vi "App - analyze RUS V6.vi"() -> ()   [LabVIEW 2021] (continued)
"z center"=0.03600000000000003+0.0040000000000000036i, "z(0)"=-0.1817049418249758+0.4229026946079033i, "radius"=0.47209629234381667}}, "timestamp(min)"=320.0, "timestamp"=timestamp(3493747021 s since 1904-01-01), "Magn Field(T)"=0.0}, {"temperature"=155.917, "lorentzian"={"A (VHz)"=0.0003600783098296233, "ω (Hz)"=667.5871571554018, "Γ (Hz)"=0.0666645074516891, "φ (rad)"=3.6415323231958747, "Q"=10014.131697278248, "Norm  Ampl"=0.03138403226728406, "z∞ (V)"=0.2616769830982948-0.40115818854601326i, "4corners"={"z (-pi/2)"=-0.37715818854601324-0.21367698309829475i, "z(inf)"=0.2616769830982948-0.40115818854601326i, "z (pi/2)"=0.4491581885460133+0.23767698309829477i, "z center"=0.03600000000000003+0.01200000000000001i, "z(0)"=-0.18967698309829473+0.4251581885460133i, "radius"=0.4707757315994221}}, "timestamp(min)"=321.33333333581686, "timestamp"=timestamp(3493747101 s since 1904-01-01), "Magn Field(T)"=0.0}, {"temperature"=155.569, "lorentzian"={"A (VHz)"=0.0003591126324986569, "ω (Hz)"=667.603372353538, "Γ (Hz)"=0.06609971655941053, "φ (rad)"=3.6523793327906917, "Q"=10099.943042168645, "Norm  Ampl"=0.03138978061501275, "z∞ (V)"=0.2681541455231212-0.4022709936013601i, "4corners"={"z (-pi/2)"=-0.3782709936013601-0.22015414552312118i, "z(inf)"=0.2681541455231212-0.4022709936013601i, "z (pi/2)"=0.45027099360136014+0.2441541455231212i, "z center"=0.03600000000000003+0.01200000000000001i, "z(0)"=-0.19615414552312116+0.4262709936013601i, "radius"=0.47488525290119155}}, "timestamp(min)"=322.6499999985099, "timestamp"=timestamp(3493747180 s since 1904-01-01), "Magn Field(T)"=0.0}, {"temperature"=155.24, "lorentzian"={"A (VHz)"=0.0003558702433597225, "ω (Hz)"=667.6196504795548, "Γ (Hz)"=0.06570935152346731, "φ (rad)"=3.666739520729764, "Q"=10160.192347068323, "Norm  Ampl"=0.03117556747840149, "z∞ (V)"=0.27385901621365416-0.39851492868577315i, "4corners"={"z (-pi/2)"=-0.37451492868577313-0.22585901621365412i, "z(inf)"=0.27385901621365416-0.39851492868577315i, "z (pi/2)"=0.4465149286857732+0.24985901621365414i, "z center"=0.03600000000000003+0.01200000000000001i, "z(0)"=-0.2018590162136541+0.4225149286857732i, "radius"=0.47444643350752763}}, "timestamp(min)"=323.9666666686535, "timestamp"=timestamp(3493747259 s since 1904-01-01), "Magn Field(T)"=0.0}, {"temperature"=154.892, "lorentzian"={"A (VHz)"=0.0003530566967995145, "ω (Hz)"=667.6345004307237, "Γ (Hz)"=0.06544080329072241, "φ (rad)"=3.6774068000638085, "Q"=10202.11346527549, "Norm  Ampl"=0.03099707161072482, "z∞ (V)"=0.27782594111484155-0.3952830971115466i, "4corners"={"z (-pi/2)"=-0.37128309711154656-0.2298259411148415i, "z(inf)"=0.27782594111484155-0.3952830971115466i, "z (pi/2)"=0.4432830971115466+0.2538259411148415i, "z center"=0.03600000000000003+0.01200000000000001i, "z(0)"=-0.20582594111484148+0.4192830971115466i, "radius"=0.4736658178387504}}, "timestamp(min)"=325.30000000447035, "timestamp"=timestamp(3493747339 s since 1904-01-01), "Magn Field(T)"=0.0}, {"temperature"=154.55, "lorentzian"={"A (VHz)"=0.00035235220794812265, "ω (Hz)"=667.6414584582035, "Γ (Hz)"=0.06583438070884551, "φ (rad)"=3.6599783805757107, "Q"=10141.227900523096, "Norm  Ampl"=0.031187058102442655, "z∞ (V)"=0.262718083957458-0.39948267452777714i, "4corners"={"z (-pi/2)"=-0.3834826745277771-0.22271808395745793i, "z(inf)"=0.262718083957458-0.39948267452777714i, "z (pi/2)"=0.4394826745277772+0.24671808395745795i, "z center"=0.028000000000000025+0.01200000000000001i, "z(0)"=-0.20671808395745792+0.42348267452777716i, "radius"=0.4737199281993453}}, "timestamp(min)"=326.6166666671634, "timestamp"=timestamp(3493747418 s since 1904-01-01), "Magn Field(T)"=0.0}, {"temperature"=154.223, "lorentzian"={"A (VHz)"=0.0003545258955251594, "ω (Hz)"=667.6596980423662, "Γ (Hz)"=0.06596121803706546, "φ (rad)"=3.6664657392703672, "Q"=10122.003776024716, "Norm  Ampl"=0.03132255223514789, "z∞ (V)"=0.2739554373795724-0.40694066198896567i, "4corners"={"z (-pi/2)"=-0.37494066198896564-0.23395543737957233i, "z(inf)"=0.2739554373795724-0.40694066198896567i, "z (pi/2)"=0.4469406619889657+0.24195543737957234i, "z center"=0.03600000000000003+0.0040000000000000036i, "z(0)"=-0.2019554373795723+0.4149406619889657i, "radius"=0.47486315697728426}}, "timestamp(min)"=327.95000000298023, "timestamp"=timestamp(3493747498 s since 1904-01-01), "Magn Field(T)"=0.0}, {"temperature"=153.877, "lorentzian"={"A (VHz)"=0.0003464844794787016, "ω (Hz)"=667.6762506062214, "Γ (Hz)"=0.06468629451459908, "φ (rad)"=3.686205850400607, "Q"=10321.757578114684, "Norm  Ampl"=0.030601207625047026, "z∞ (V)"=0.2810920510849647-0.3926307234080894i, "4corners"={"z (-pi/2)"=-0.3686307234080894-0.2330920510849647i, "z(inf)"=0.2810920510849647-0.3926307234080894i, "z (pi/2)"=0.44063072340808945+0.2570920510849647i, "z center"=0.03600000000000003+0.01200000000000001i, "z(0)"=-0.20909205108496468+0.41663072340808943i, "radius"=0.47307096278548816}}, "timestamp(min)"=329.26666666567326, "timestamp"=timestamp(3493747577 s since 1904-01-01), "Magn Field(T)"=0.0}, {"temperature"=153.533, "lorentzian"={"A (VHz)"=0.00034529942679625386, "ω (Hz)"=667.6919916866713, "Γ (Hz)"=0.06439844993865426, "φ (rad)"=3.697376351094415, "Q"=10368.137623230254, "Norm  Ampl"=0.030502173386016206, "z∞ (V)"=0.28590085026076295-0.3903576087759872i, "4corners"={"z (-pi/2)"=-0.36635760877598716-0.2379008502607629i, "z(inf)"=0.28590085026076295-0.3903576087759872i, "z (pi/2)"=0.43835760877598723+0.26190085026076293i, "z center"=0.03600000000000003+0.01200000000000001i, "z(0)"=-0.2139008502607629+0.4143576087759872i, "radius"=0.47364763305751106}}, "timestamp(min)"=330.58333333581686, "timestamp"=timestamp(3493747656 s since 1904-01-01), "Magn Field(T)"=0.0}, {"temperature"=153.206, "lorentzian"={"A (VHz)"=0.00034827333081709075, "ω (Hz)"=667.704330610667, "Γ (Hz)"=0.0656929969706585, "φ (rad)"=3.67323809413097, "Q"=10164.010798729341, "Norm  Ampl"=0.03128951043987482, "z∞ (V)"=0.2774609121600786-0.4065574132803119i, "4corners"={"z (-pi/2)"=-0.3745574132803119-0.23746091216007859i, "z(inf)"=0.2774609121600786-0.4065574132803119i, "z (pi/2)"=0.44655741328031195+0.2454609121600786i, "z center"=0.03600000000000003+0.0040000000000000036i, "z(0)"=-0.20546091216007856+0.4145574132803119i, "radius"=0.4762990255087638}}, "timestamp(min)"=331.91666666418314, "timestamp"=timestamp(3493747736 s since 1904-01-01), "Magn Field(T)"=0.0}, {"temperature"=152.863, "lorentzian"={"A (VHz)"=0.0003372130117361326, "ω (Hz)"=667.7178274337781, "Γ (Hz)"=0.06419396759064425, "φ (rad)"=3.6582012443053293, "Q"=10401.566572294132, "Norm  Ampl"=0.03048428381427238, "z∞ (V)"=0.2625583169568325-0.40090583410884956i, "4corners"={"z (-pi/2)"=-0.38490583410884954-0.2225583169568325i, "z(inf)"=0.2625583169568325-0.40090583410884956i, "z (pi/2)"=0.4409058341088496+0.24655831695683253i, "z center"=0.028000000000000025+0.01200000000000001i, "z(0)"=-0.2065583169568325+0.4249058341088496i, "radius"=0.47487770203995333}}, "timestamp(min)"=333.23333333432674, "timestamp"=timestamp(3493747815 s since 1904-01-01), "Magn Field(T)"=0.0}, {"temperature"=152.533, "lorentzian"={"A (VHz)"=0.0003397272875597955, "ω (Hz)"=667.7315679125422, "Γ (Hz)"=0.06505456301107017, "φ (rad)"=3.657146799356104, "Q"=10264.17728451909, "Norm  Ampl"=0.030891975244662705, "z∞ (V)"=0.2701153266514513-0.409139744947861i, "4corners"={"z (-pi/2)"=-0.37713974494786096-0.23011532665145132i, "z(inf)"=0.2701153266514513-0.409139744947861i, "z (pi/2)"=0.449139744947861+0.23811532665145133i, "z center"=0.03600000000000003+0.0040000000000000036i, "z(0)"=-0.1981153266514513+0.417139744947861i, "radius"=0.47486254329932087}}, "timestamp(min)"=334.5666666701436, "timestamp"=timestamp(3493747895 s since 1904-01-01), "Magn Field(T)"=0.0}, {"temperature"=152.199, "lorentzian"={"A (VHz)"=0.00033208611082412016, "ω (Hz)"=667.7469406174972, "Γ (Hz)"=0.0635522497688255, "φ (rad)"=3.6578539107424763, "Q"=10507.054322175223, "Norm  Ampl"=0.029929110405591684, "z∞ (V)"=0.260469665044331-0.3975602279620725i, "4corners"={"z (-pi/2)"=-0.3815602279620725-0.22046966504433094i, "z(inf)"=0.260469665044331-0.3975602279620725i, "z (pi/2)"=0.43756022796207256+0.24446966504433096i, "z center"=0.028000000000000025+0.01200000000000001i, "z(0)"=-0.20446966504433092+0.42156022796207254i, "radius"=0.47093707169235277}}, "timestamp(min)"=335.8833333328366, "timestamp"=timestamp(3493747974 s since 1904-01-01), "Magn Field(T)"=0.0}, {"temperature"=151.853, "lorentzian"={"A (VHz)"=0.0003330053751699988, "ω (Hz)"=667.7605274396784, "Γ (Hz)"=0.06353834993859891, "φ (rad)"=3.6627469445655536, "Q"=10509.56671183588, "Norm  Ampl"=0.030019978731297435, "z∞ (V)"=0.27123419681365424-0.3977474706761259i, "4corners"={"z (-pi/2)"=-0.3737474706761259-0.22323419681365422i, "z(inf)"=0.27123419681365424-0.3977474706761259i, "z (pi/2)"=0.44574747067612597+0.24723419681365424i, "z center"=0.03600000000000003+0.01200000000000001i, "z(0)"=-0.1992341968136542+0.42174747067612595i, "radius"=0.4724702287721923}}, "timestamp(min)"=337.20000000298023, "timestamp"=timestamp(3493748053 s since 1904-01-01), "Magn Field(T)"=0.0}, {"temperature"=151.527, "lorentzian"={"A (VHz)"=0.0003295932580058115, "ω (Hz)"=667.772514287168, "Γ (Hz)"=0.0630130233034684, "φ (rad)"=3.647573399320795, "Q"=10597.373039398539, "Norm  Ampl"=0.02979783733634646, "z∞ (V)"=0.26519047368720017-0.40163124455846033i, "4corners"={"z (-pi/2)"=-0.3776312445584603-0.2171904736872001i, "z(inf)"=0.26519047368720017-0.40163124455846033i, "z (pi/2)"=0.4496312445584604+0.24119047368720012i, "z center"=0.03600000000000003+0.01200000000000001i, "z(0)"=-0.19319047368720008+0.42563124455846035i, "radius"=0.4728837909084472}}, "timestamp(min)"=338.5333333313465, "timestamp"=timestamp(3493748133 s since 1904-01-01), "Magn Field(T)"=0.0}, {"temperature"=151.178, "lorentzian"={"A (VHz)"=0.00033462286002910205, "ω (Hz)"=667.7857246989796, "Γ (Hz)"=0.0642850672644637, "φ (rad)"=3.640302404861034, "Q"=10387.882491462002, "Norm  Ampl"=0.030484425861645383, "z∞ (V)"=0.262809790264348-0.41244874015600735i, "4corners"={"z (-pi/2)"=-0.3804487401560073-0.22280979026434794i, "z(inf)"=0.262809790264348-0.41244874015600735i, "z (pi/2)"=0.4524487401560074+0.23080979026434795i, "z center"=0.03600000000000003+0.0040000000000000036i, "z(0)"=-0.1908097902643479+0.42044874015600736i, "radius"=0.47420695285632747}}, "timestamp(min)"=339.8500000014901, "timestamp"=timestamp(3493748212 s since 1904-01-01), "Magn Field(T)"=0.0}, {"temperature"=150.857, "lorentzian"={"A (VHz)"=0.00032734963388068015, "ω (Hz)"=667.7975632145829, "Γ (Hz)"=0.06366705232811726, "φ (rad)"=3.6387119410670934, "Q"=10488.903424851407, "Norm  Ampl"=0.030098814806053722, "z∞ (V)"=0.26145395936377014-0.4035313222431252i, "4corners"={"z (-pi/2)"=-0.3795313222431252-0.2134539593637701i, "z(inf)"=0.26145395936377014-0.4035313222431252i, "z (pi/2)"=0.45153132224312525+0.23745395936377012i, "z center"=0.03600000000000003+0.01200000000000001i, "z(0)"=-0.18945395936377007+0.42753132224312523i, "radius"=0.47275338978998394}}, "timestamp(min)"=341.16666666418314, "timestamp"=timestamp(3493748291 s since 1904-01-01), "Magn Field(T)"=0.0}, {"temperature"=150.523, "lorentzian"={"A (VHz)"=0.00032705985282191106, "ω (Hz)"=667.8113824108048, "Γ (Hz)"=0.06350429444344641, "φ (rad)"=3.628258749601216, "Q"=10516.003496511918, "Norm  Ampl"=0.030253572882116685, "z∞ (V)"=0.2588044806232093-0.4170902860768382i, "4corners"={"z (-pi/2)"=-0.38509028607683815-0.21880448062320929i, "z(inf)"=0.2588044806232093-0.4170902860768382i, "z (pi/2)"=0.4570902860768382+0.2268044806232093i, "z center"=0.03600000000000003+0.0040000000000000036i, "z(0)"=-0.18680448062320926+0.4250902860768382i, "radius"=0.4764020000105494}}, "timestamp(min)"=342.5, "timestamp"=timestamp(3493748371 s since 1904-01-01), "Magn Field(T)"=0.0}, {"temperature"=150.18, "lorentzian"={"A (VHz)"=0.00031895506176438625, "ω (Hz)"=667.8259629307869, "Γ (Hz)"=0.062260001868224786, "φ (rad)"=3.65113689178434, "Q"=10726.404479464378, "Norm  Ampl"=0.029328326932120865, "z∞ (V)"=0.265774401546258-0.3992216215165581i, "4corners"={"z (-pi/2)"=-0.3752216215165581-0.2177744015462579i, "z(inf)"=0.265774401546258-0.3992216215165581i, "z (pi/2)"=0.44722162151655814+0.24177440154625793i, "z center"=0.03600000000000003+0.01200000000000001i, "z(0)"=-0.19377440154625789+0.4232216215165581i, "radius"=0.4710620952790071}}, "timestamp(min)"=343.8166666701436, "timestamp"=timestamp(3493748450 s since 1904-01-01), "Magn Field(T)"=0.0}, {"temperature"=149.856, "lorentzian"={"A (VHz)"=0.0003180644929081725, "ω (Hz)"=667.8339870162451, "Γ (Hz)"=0.0626104577337908, "φ (rad)"=3.6118990790654046, "Q"=10666.49264657613, "Norm  Ampl"=0.029413288089057528, "z∞ (V)"=0.24888631848769124-0.4147778331974934i, "4corners"={"z (-pi/2)"=-0.38277783319749337-0.2088863184876912i, "z(inf)"=0.24888631848769124-0.4147778331974934i, "z (pi/2)"=0.45477783319749343+0.21688631848769122i, "z center"=0.03600000000000003+0.0040000000000000036i, "z(0)"=-0.17688631848769118+0.4227778331974934i, "radius"=0.46978235192143003}}, "timestamp(min)"=345.1499999985099, "timestamp"=timestamp(3493748530 s since 1904-01-01), "Magn Field(T)"=0.0}, {"temperature"=149.518, "lorentzian"={"A (VHz)"=0.0003207517090712809, "ω (Hz)"=667.846314585591, "Γ (Hz)"=0.06260199340788268, "φ (rad)"=3.6167471348240188, "Q"=10668.13176753406, "Norm  Ampl"=0.02952394034540045, "z∞ (V)"=0.2437517373853843-0.4153690591599955i, "4corners"={"z (-pi/2)"=-0.3913690591599955-0.21175173738538428i, "z(inf)"=0.2437517373853843-0.4153690591599955i, "z (pi/2)"=0.44736905915999553+0.21975173738538428i, "z center"=0.028000000000000025+0.0040000000000000036i, "z(0)"=-0.18775173738538425+0.4233690591599955i, "radius"=0.47161342216433116}}, "timestamp(min)"=346.4666666686535, "timestamp"=timestamp(3493748609 s since 1904-01-01), "Magn Field(T)"=0.0}, {"temperature"=149.197, "lorentzian"={"A (VHz)"=0.0003234783703784625, "ω (Hz)"=667.8533606686503, "Γ (Hz)"=0.06359946620713222, "φ (rad)"=3.6201299277993155, "Q"=10500.927138186506, "Norm  Ampl"=0.030006919790938662, "z∞ (V)"=0.24526006219172095-0.4148120903216504i, "4corners"={"z (-pi/2)"=-0.3908120903216504-0.21326006219172092i, "z(inf)"=0.24526006219172095-0.4148120903216504i, "z (pi/2)"=0.4468120903216504+0.22126006219172092i, "z center"=0.028000000000000025+0.0040000000000000036i, "z(0)"=-0.1892600621917209+0.4228120903216504i, "radius"=0.4718108748462043}}, "timestamp(min)"=347.7833333313465, "timestamp"=timestamp(3493748688 s since 1904-01-01), "Magn Field(T)"=0.0}, {"temperature"=148.854, "lorentzian"={"A (VHz)"=0.00031661202440796217, "ω (Hz)"=667.8697794122957, "Γ (Hz)"=0.06259438686006111, "φ (rad)"=3.6381230108136604, "Q"=10669.803043289106, "Norm  Ampl"=0.029435172808309772, "z∞ (V)"=0.26001787794724807-0.4094652256080112i, "4corners"={"z (-pi/2)"=-0.37746522560801116-0.22001787794724803i, "z(inf)"=0.26001787794724807-0.4094652256080112i, "z (pi/2)"=0.4494652256080112+0.22801787794724804i, "z center"=0.03600000000000003+0.0040000000000000036i, "z(0)"=-0.188017877947248+0.4174652256080112i, "radius"=0.4702525942800015}}, "timestamp(min)"=349.1166666671634, "timestamp"=timestamp(3493748768 s since 1904-01-01), "Magn Field(T)"=0.0}, {"temperature"=148.52, "lorentzian"={"A (VHz)"=0.00034844810283746436, "ω (Hz)"=667.8814288240087, "Γ (Hz)"=0.07085049634721703, "φ (rad)"=3.629245704211228, "Q"=9426.63020384391, "Norm  Ampl"=0.03241702676273373, "z∞ (V)"=0.3143827067821342-0.42420796332950217i, "4corners"={"z (-pi/2)"=-0.3042079633295022-0.23438270678213424i, "z(inf)"=0.3143827067821342-0.42420796332950217i, "z (pi/2)"=0.5042079633295021+0.1943827067821342i, "z center"=0.09999999999999998-0.020000000000000018i, "z(0)"=-0.11438270678213425+0.38420796332950213i, "radius"=0.45754127965268737}}, "timestamp(min)"=350.433333337307, "timestamp"=timestamp(3493748847 s since 1904-01-01), "Magn Field(T)"=0.0}, {"temperature"=148.201, "lorentzian"={"A (VHz)"=0.0003073002085522271, "ω (Hz)"=667.8943565204472, "Γ (Hz)"=0.061248128995911304, "φ (rad)"=3.6528288778442097, "Q"=10904.730764347649, "Norm  Ampl"=0.02830335435436209, "z∞ (V)"=0.2620898411257922-0.39102451059062343i, "4corners"={"z (-pi/2)"=-0.3670245105906234-0.21408984112579216i, "z(inf)"=0.2620898411257922-0.39102451059062343i, "z (pi/2)"=0.4390245105906235+0.23808984112579218i, "z center"=0.03600000000000003+0.01200000000000001i, "z(0)"=-0.19008984112579214+0.41502451059062345i, "radius"=0.46210969736318835}}, "timestamp(min)"=351.75, "timestamp"=timestamp(3493748926 s since 1904-01-01), "Magn Field(T)"=0.0}, {"temperature"=147.858, "lorentzian"={"A (VHz)"=0.00031057161752807115, "ω (Hz)"=667.9070637171257, "Γ (Hz)"=0.0614808732740524, "φ (rad)"=3.6653109549557077, "Q"=10863.656095773309, "Norm  Ampl"=0.028670623619861096, "z∞ (V)"=0.26921528643990444-0.3998292473492588i, "4corners"={"z (-pi/2)"=-0.36782924734925876-0.2292152864399044i, "z(inf)"=0.26921528643990444-0.3998292473492588i, "z (pi/2)"=0.4398292473492588+0.23721528643990442i, "z center"=0.03600000000000003+0.0040000000000000036i, "z(0)"=-0.19721528643990438+0.4078292473492588i, "radius"=0.46633403354667935}}, "timestamp(min)"=353.08333333581686, "timestamp"=timestamp(3493749006 s since 1904-01-01), "Magn Field(T)"=0.0}, {"temperature"=147.54, "lorentzian"={"A (VHz)"=0.0003460988710122296, "ω (Hz)"=667.9189901657315, "Γ (Hz)"=0.06935167471007338, "φ (rad)"=3.6631658495938564, "Q"=9630.899224250685, "Norm  Ampl"=0.031501878165273896, "z∞ (V)"=0.3263196407566756-0.4138372889156103i, "4corners"={"z (-pi/2)"=-0.2938372889156103-0.24631964075667562i, "z(inf)"=0.3263196407566756-0.4138372889156103i, "z (pi/2)"=0.49383728891561024+0.20631964075667558i, "z center"=0.09999999999999998-0.020000000000000018i, "z(0)"=-0.12631964075667562+0.37383728891561024i, "radius"=0.4542338493910692}}, "timestamp(min)"=354.3999999985099, "timestamp"=timestamp(3493749085 s since 1904-01-01), "Magn Field(T)"=0.0}, {"temperature"=147.208, "lorentzian"={"A (VHz)"=0.0003065721569098357, "ω (Hz)"=667.9290708716037, "Γ (Hz)"=0.06055692944372653, "φ (rad)"=3.621241049474215, "Q"=11029.771109717298, "Norm  Ampl"=0.028232663149197763, "z∞ (V)"=0.2591438369751396-0.4096076829648885i, "4corners"={"z (-pi/2)"=-0.36960768296488844-0.21114383697513955i, "z(inf)"=0.2591438369751396-0.4096076829648885i, "z (pi/2)"=0.4576076829648885+0.21914383697513956i, "z center"=0.04400000000000004+0.0040000000000000036i, "z(0)"=-0.17114383697513952+0.4176076829648885i, "radius"=0.46621688729170796}}, "timestamp(min)"=355.73333333432674, "timestamp"=timestamp(3493749165 s since 1904-01-01), "Magn Field(T)"=0.0}, {"temperature"=146.868, "lorentzian"={"A (VHz)"=0.0002962982041096755, "ω (Hz)"=667.9412342117888, "Γ (Hz)"=0.05902727065464663, "φ (rad)"=3.6161204795961823, "Q"=11315.807537836894, "Norm  Ampl"=0.02764749945528269, "z∞ (V)"=0.25001385682058386-0.41263263972332964i, "4corners"={"z (-pi/2)"=-0.3806326397233296-0.21001385682058385i, "z(inf)"=0.25001385682058386-0.41263263972332964i, "z (pi/2)"=0.4526326397233297+0.21801385682058386i, "z center"=0.03600000000000003+0.0040000000000000036i, "z(0)"=-0.17801385682058382+0.42063263972332965i, "radius"=0.4683851912625453}}, "timestamp(min)"=357.05000000447035, "timestamp"=timestamp(3493749244 s since 1904-01-01), "Magn Field(T)"=0.0}, {"temperature"=146.551, "lorentzian"={"A (VHz)"=0.0003678362542505415, "ω (Hz)"=667.9478689614617, "Γ (Hz)"=0.07421100844783732, "φ (rad)"=3.537703817949713, "Q"=9000.65748912387, "Norm  Ampl"=0.03401887709945447, "z∞ (V)"=0.2848689640299755-0.4429122066264123i, "4corners"={"z (-pi/2)"=-0.3149122066264123-0.19686896402997556i, "z(inf)"=0.2848689640299755-0.4429122066264123i, "z (pi/2)"=0.5309122066264123+0.15686896402997552i, "z center"=0.10799999999999998-0.020000000000000018i, "z(0)"=-0.06886896402997555+0.40291220662641225i, "radius"=0.45840742244280686}}, "timestamp(min)"=358.3666666671634, "timestamp"=timestamp(3493749323 s since 1904-01-01), "Magn Field(T)"=0.0}, {"temperature"=146.222, "lorentzian"={"A (VHz)"=0.00029746239323954273, "ω (Hz)"=667.9595344300756, "Γ (Hz)"=0.058724356418033107, "φ (rad)"=3.564390599368359, "Q"=11374.488801123041, "Norm  Ampl"=0.02745634019372911, "z∞ (V)"=0.2278405107541988-0.42237602693380516i, "4corners"={"z (-pi/2)"=-0.39037602693380513-0.18784051075419878i, "z(inf)"=0.2278405107541988-0.42237602693380516i, "z (pi/2)"=0.4623760269338052+0.19584051075419878i, "z center"=0.03600000000000003+0.0040000000000000036i, "z(0)"=-0.15584051075419875+0.43037602693380517i, "radius"=0.4675460382788938}}, "timestamp(min)"=359.70000000298023, "timestamp"=timestamp(3493749403 s since 1904-01-01), "Magn Field(T)"=0.0}, {"temperature"=145.898, "lorentzian"={"A (VHz)"=0.00029752632281150864, "ω (Hz)"=667.9715429031386, "Γ (Hz)"=0.05899742914650107, "φ (rad)"=3.585419866476969, "Q"=11322.044919015825, "Norm  Ampl"=0.02760993852940348, "z∞ (V)"=0.23695249170078814-0.4186446250695427i, "4corners"={"z (-pi/2)"=-0.38664462506954267-0.1969524917007881i, "z(inf)"=0.23695249170078814-0.4186446250695427i, "z (pi/2)"=0.45864462506954273+0.2049524917007881i, "z center"=0.03600000000000003+0.0040000000000000036i, "z(0)"=-0.16495249170078807+0.4266446250695427i, "radius"=0.4679854517193132}}, "timestamp(min)"=361.01666666567326, "timestamp"=timestamp(3493749482 s since 1904-01-01), "Magn Field(T)"=0.0}, {"temperature"=145.567, "lorentzian"={"A (VHz)"=0.0002927870548625147, "ω (Hz)"=667.98053690319, "Γ (Hz)"=0.058207561543709985, "φ (rad)"=3.568654044791983, "Q"=11475.8378325397, "Norm  Ampl"=0.027295941833282978, "z∞ (V)"=0.23023459431411045-0.422824393221578i, "4corners"={"z (-pi/2)"=-0.39082439322157797-0.1902345943141104i, "z(inf)"=0.23023459431411045-0.422824393221578i, "z (pi/2)"=0.46282439322157803+0.19823459431411042i, "z center"=0.03600000000000003+0.0040000000000000036i, "z(0)"=-0.15823459431411038+0.430824393221578i, "radius"=0.46894151050779803}}, "timestamp(min)"=362.33333333581686, "timestamp"=timestamp(3493749561 s since 1904-01-01), "Magn Field(T)"=0.0}, {"temperature"=145.231, "lorentzian"={"A (VHz)"=0.000290993922150055, "ω (Hz)"=667.9933159378816, "Γ (Hz)"=0.05804473579725992, "φ (rad)"=3.5990724327102, "Q"=11508.249745008145, "Norm  Ampl"=0.027099557940129443, "z∞ (V)"=0.24221270056849373-0.41486433557329433i, "4corners"={"z (-pi/2)"=-0.3828643355732943-0.2022127005684937i, "z(inf)"=0.24221270056849373-0.41486433557329433i, "z (pi/2)"=0.45486433557329436+0.2102127005684937i, "z center"=0.03600000000000003+0.0040000000000000036i, "z(0)"=-0.17021270056849366+0.42286433557329434i, "radius"=0.4668736547407752}}, "timestamp(min)"=363.66666666418314, "timestamp"=timestamp(3493749641 s since 1904-01-01), "Magn Field(T)"=0.0}, {"temperature"=144.914, "lorentzian"={"A (VHz)"=0.00032066513695734307, "ω (Hz)"=668.0042574571033, "Γ (Hz)"=0.06909736501950893, "φ (rad)"=3.5444896463253777, "Q"=9667.579324747032, "Norm  Ampl"=0.030135599602355533, "z∞ (V)"=0.2790009768476864-0.4132108370623837i, "4corners"={"z (-pi/2)"=-0.2932108370623837-0.1830009768476864i, "z(inf)"=0.2790009768476864-0.4132108370623837i, "z (pi/2)"=0.5092108370623837+0.15900097684768638i, "z center"=0.10799999999999998-0.01200000000000001i, "z(0)"=-0.06300097684768641+0.3892108370623837i, "radius"=0.43613239946048676}}, "timestamp(min)"=364.98333333432674, "timestamp"=timestamp(3493749720 s since 1904-01-01), "Magn Field(T)"=0.0}, {"temperature"=144.597, "lorentzian"={"A (VHz)"=0.000274526279485729, "ω (Hz)"=668.0186275854775, "Γ (Hz)"=0.0565158521956909, "φ (rad)"=3.5988418696111295, "Q"=11820.022199654828, "Norm  Ampl"=0.02640927490968859, "z∞ (V)"=0.2502997912176008-0.40728516329633496i, "4corners"={"z (-pi/2)"=-0.37528516329633493-0.19429979121760077i, "z(inf)"=0.2502997912176008-0.40728516329633496i, "z (pi/2)"=0.463285163296335+0.2182997912176008i, "z center"=0.04400000000000004+0.01200000000000001i, "z(0)"=-0.16229979121760074+0.431285163296335i, "radius"=0.4672896874711231}}, "timestamp(min)"=366.3166666701436, "timestamp"=timestamp(3493749800 s since 1904-01-01), "Magn Field(T)"=0.0}, {"temperature"=144.27, "lorentzian"={"A (VHz)"=0.00030202505213323613, "ω (Hz)"=668.0261021371313, "Γ (Hz)"=0.06388234206541538, "φ (rad)"=3.575176862528663, "Q"=10457.132292568016, "Norm  Ampl"=0.028924959474196967, "z∞ (V)"=0.29822672487411456-0.4388867888945171i, "4corners"={"z (-pi/2)"=-0.3028867888945171-0.2182267248741146i, "z(inf)"=0.29822672487411456-0.4388867888945171i, "z (pi/2)"=0.518886788894517+0.16222672487411455i, "z center"=0.10799999999999998-0.028000000000000025i, "z(0)"=-0.08222672487411459+0.38288678889451705i, "radius"=0.45278489390038124}}, "timestamp(min)"=367.6333333328366, "timestamp"=timestamp(3493749879 s since 1904-01-01), "Magn Field(T)"=0.0}, {"temperature"=143.94, "lorentzian"={"A (VHz)"=0.0003016721792558354, "ω (Hz)"=668.038205785295, "Γ (Hz)"=0.0632442645829743, "φ (rad)"=3.573907501497747, "Q"=10562.826687767896, "Norm  Ampl"=0.02871544420979473, "z∞ (V)"=0.2902309860102974-0.43226782142765685i, "4corners"={"z (-pi/2)"=-0.31226782142765686-0.2102309860102974i, "z(inf)"=0.2902309860102974-0.43226782142765685i, "z (pi/2)"=0.5122678214276568+0.17023098601029737i, "z center"=0.09999999999999998-0.020000000000000018i, "z(0)"=-0.09023098601029741+0.3922678214276568i, "radius"=0.4540402896474676}}, "timestamp(min)"=368.95000000298023, "timestamp"=timestamp(3493749958 s since 1904-01-01), "Magn Field(T)"=0.0}, {"temperature"=143.619, "lorentzian"={"A (VHz)"=0.00029228013832460813, "ω (Hz)"=668.0502969770072, "Γ (Hz)"=0.06173081228691563, "φ (rad)"=3.5741941798931562, "Q"=10821.991032160873, "Norm  Ampl"=0.02813796545614369, "z∞ (V)"=0.29109410409542597-0.4338264793501994i, "4corners"={"z (-pi/2)"=-0.3138264793501994-0.211094104095426i, "z(inf)"=0.29109410409542597-0.4338264793501994i, "z (pi/2)"=0.5138264793501994+0.17109410409542597i, "z center"=0.09999999999999998-0.020000000000000018i, "z(0)"=-0.09109410409542601+0.3938264793501994i, "radius"=0.45581719102225016}}, "timestamp(min)"=370.2833333313465, "timestamp"=timestamp(3493750038 s since 1904-01-01), "Magn Field(T)"=0.0}, {"temperature"=143.299, "lorentzian"={"A (VHz)"=0.00029997840689162354, "ω (Hz)"=668.0581032164006, "Γ (Hz)"=0.062376618472958036, "φ (rad)"=3.5461493505054786, "Q"=10710.072452966042, "Norm  Ampl"=0.028666591404283952, "z∞ (V)"=0.2808930017905096-0.4424746085981441i, "4corners"={"z (-pi/2)"=-0.3224746085981441-0.2008930017905096i, "z(inf)"=0.2808930017905096-0.4424746085981441i, "z (pi/2)"=0.522474608598144+0.16089300179050955i, "z center"=0.09999999999999998-0.020000000000000018i, "z(0)"=-0.0808930017905096+0.40247460859814405i, "radius"=0.4595727069865402}}, "timestamp(min)"=371.6000000014901, "timestamp"=timestamp(3493750117 s since 1904-01-01), "Magn Field(T)"=0.0}, {"temperature"=142.977, "lorentzian"={"A (VHz)"=0.0002958401330853481, "ω (Hz)"=668.0629833326522, "Γ (Hz)"=0.06019497441453552, "φ (rad)"=3.465579755013286, "Q"=11098.3182538131, "Norm  Ampl"=0.028649324626753108, "z∞ (V)"=0.25951558280354314-0.4711806111087101i, "4corners"={"z (-pi/2)"=-0.3431806111087101-0.1715155828035432i, "z(inf)"=0.25951558280354314-0.4711806111087101i, "z (pi/2)"=0.5591806111087101+0.13151558280354317i, "z center"=0.10799999999999998-0.020000000000000018i, "z(0)"=-0.0435155828035432+0.4311806111087101i, "radius"=0.4759421347944795}}, "timestamp(min)"=372.933333337307, "timestamp"=timestamp(3493750197 s since 1904-01-01), "Magn Field(T)"=0.0}, {"temperature"=142.653, "lorentzian"={"A (VHz)"=0.00029958880555415376, "ω (Hz)"=668.0682070709669, "Γ (Hz)"=0.05852985303538896, "φ (rad)"=3.4121450113994722, "Q"=11414.144618935437, "Norm  Ampl"=0.028896814733003002, "z∞ (V)"=0.23195096941323312-0.4957511926447197i, "4corners"={"z (-pi/2)"=-0.3757511926447197-0.15195096941323316i, "z(inf)"=0.23195096941323312-0.4957511926447197i, "z (pi/2)"=0.5757511926447196+0.11195096941323313i, "z center"=0.09999999999999998-0.020000000000000018i, "z(0)"=-0.031950969413233166+0.45575119264471964i, "radius"=0.49371070034177417}}, "timestamp(min)"=374.25, "timestamp"=timestamp(3493750276 s since 1904-01-01), "Magn Field(T)"=0.0}, {"temperature"=142.336, "lorentzian"={"A (VHz)"=0.00028796078361817087, "ω (Hz)"=668.0806358264088, "Γ (Hz)"=0.060482065205570014, "φ (rad)"=3.4662667178116315, "Q"=11045.929624851546, "Norm  Ampl"=0.028038898474014137, "z∞ (V)"=0.1918852558397877-0.4353699046115305i, "4corners"={"z (-pi/2)"=-0.3953699046115305-0.14388525583978765i, "z(inf)"=0.1918852558397877-0.4353699046115305i, "z (pi/2)"=0.48336990461153057+0.15188525583978765i, "z center"=0.04400000000000004+0.0040000000000000036i, "z(0)"=-0.10388525583978761+0.44336990461153053i, "radius"=0.46359029538283575}}, "timestamp(min)"=375.5666666701436, "timestamp"=timestamp(3493750355 s since 1904-01-01), "Magn Field(T)"=0.0}, {"temperature"=142.011, "lorentzian"={"A (VHz)"=0.00020384182688968917, "ω (Hz)"=668.0819765634108, "Γ (Hz)"=0.04774194369786063, "φ (rad)"=3.304155086769557, "Q"=13993.606560960949, "Norm  Ampl"=0.019755706356117814, "z∞ (V)"=0.1269727530950284-0.30834623962894i, "4corners"={"z (-pi/2)"=-0.3483462396289399+0.033027246904971636i, "z(inf)"=0.1269727530950284-0.30834623962894i, "z (pi/2)"=0.46834623962894+0.16697275309502832i, "z center"=0.06000000000000005+0.09999999999999998i, "z(0)"=-0.006972753095028289+0.50834623962894i, "radius"=0.4138018862646995}}, "timestamp(min)"=376.8999999985099, "timestamp"=timestamp(3493750435 s since 1904-01-01), "Magn Field(T)"=0.0}, {"temperature"=141.704, "lorentzian"={"A (VHz)"=0.00018454280661533404, "ω (Hz)"=668.0941556665481, "Γ (Hz)"=0.043408963253834025, "φ (rad)"=3.326551417209295, "Q"=15390.695966634028, "Norm  Ampl"=0.018129442934359474, "z∞ (V)"=0.13680702541464312-0.3105194602697091i, "4corners"={"z (-pi/2)"=-0.35051946026970904+0.023192974585356907i, "z(inf)"=0.13680702541464312-0.3105194602697091i, "z (pi/2)"=0.47051946026970914+0.17680702541464305i, "z center"=0.06000000000000005+0.09999999999999998i, "z(0)"=-0.016807025414643018+0.5105194602697091i, "radius"=0.41764284551896597}}, "timestamp(min)"=378.2166666686535, "timestamp"=timestamp(3493750514 s since 1904-01-01), "Magn Field(T)"=0.0}, {"temperature"=141.376, "lorentzian"={"A (VHz)"=0.00028130524898672764, "ω (Hz)"=668.1086689007784, "Γ (Hz)"=0.06027656553026599, "φ (rad)"=3.5603153889649946, "Q"=11084.053363413823, "Norm  Ampl"=0.027771354404382022, "z∞ (V)"=0.22333088410204752-0.41692908701689824i, "4corners"={"z (-pi/2)"=-0.3849290870168982-0.18333088410204748i, "z(inf)"=0.22333088410204752-0.41692908701689824i, "z (pi/2)"=0.45692908701689827+0.1913308841020475i, "z center"=0.03600000000000003+0.0040000000000000036i, "z(0)"=-0.15133088410204745+0.42492908701689824i, "radius"=0.46073219600472276}}, "timestamp(min)"=379.5333333313465, "timestamp"=timestamp(3493750593 s since 1904-01-01), "Magn Field(T)"=0.0}, {"temperature"=141.051, "lorentzian"={"A (VHz)"=0.00027783839005807436, "ω (Hz)"=668.1154417247612, "Γ (Hz)"=0.060075142724278496, "φ (rad)"=3.550923868112156, "Q"=11121.329245793902, "Norm  Ampl"=0.02805459737049152, "z∞ (V)"=0.2218608021994267-0.4244122752424841i, "4corners"={"z (-pi/2)"=-0.39241227524248407-0.18186080219942666i, "z(inf)"=0.2218608021994267-0.4244122752424841i, "z (pi/2)"=0.46441227524248413+0.18986080219942666i, "z center"=0.03600000000000003+0.0040000000000000036i, "z(0)"=-0.14986080219942663+0.4324122752424841i, "radius"=0.46699177227511873}}, "timestamp(min)"=380.8666666671634, "timestamp"=timestamp(3493750673 s since 1904-01-01), "Magn Field(T)"=0.0}, {"temperature"=140.75, "lorentzian"={"A (VHz)"=0.0002798594927047442, "ω (Hz)"=668.1232509827006, "Γ (Hz)"=0.06020636751341944, "φ (rad)"=3.589486639506487, "Q"=11097.219091216259, "Norm  Ampl"=0.02801454666328137, "z∞ (V)"=0.23751040935297757-0.415411185122238i, "4corners"={"z (-pi/2)"=-0.383411185122238-0.19751040935297753i, "z(inf)"=0.23751040935297757-0.415411185122238i, "z (pi/2)"=0.45541118512223805+0.20551040935297754i, "z center"=0.03600000000000003+0.0040000000000000036i, "z(0)"=-0.1655104093529775+0.423411185122238i, "radius"=0.4653087010611824}}, "timestamp(min)"=382.183333337307, "timestamp"=timestamp(3493750752 s since 1904-01-01), "Magn Field(T)"=0.0}, {"temperature"=140.423, "lorentzian"={"A (VHz)"=0.00024889265270781267, "ω (Hz)"=668.1252877234232, "Γ (Hz)"=0.052615522870268064, "φ (rad)"=3.5061445309278896, "Q"=12698.254265586076, "Norm  Ampl"=0.024701401159263687, "z∞ (V)"=0.20338039069891614-0.4346179846696116i, "4corners"={"z (-pi/2)"=-0.4026179846696116-0.1633803906989161i, "z(inf)"=0.20338039069891614-0.4346179846696116i, "z (pi/2)"=0.47461798466961164+0.1713803906989161i, "z center"=0.03600000000000003+0.0040000000000000036i, "z(0)"=-0.13138039069891608+0.4426179846696116i, "radius"=0.46946984106133316}}, "timestamp(min)"=383.51666666567326, "timestamp"=timestamp(3493750832 s since 1904-01-01), "Magn Field(T)"=0.0}, {"temperature"=140.113, "lorentzian"={"A (VHz)"=0.00020276514598236694, "ω (Hz)"=668.1324581018087, "Γ (Hz)"=0.04850993210200322, "φ (rad)"=3.38998781117471, "Q"=13773.106437191202, "Norm  Ampl"=0.020213477220847074, "z∞ (V)"=0.1544420499298441-0.31189851601928653i, "4corners"={"z (-pi/2)"=-0.35189851601928646-0.010442049929844072i, "z(inf)"=0.1544420499298441-0.31189851601928653i, "z (pi/2)"=0.45589851601928655+0.194442049929844i, "z center"=0.052000000000000046+0.09199999999999997i, "z(0)"=-0.050442049929843996+0.4958985160192865i, "radius"=0.4166873946214482}}, "timestamp(min)"=384.83333333581686, "timestamp"=timestamp(3493750911 s since 1904-01-01), "Magn Field(T)"=0.0}, {"temperature"=139.803, "lorentzian"={"A (VHz)"=0.00027477475506784184, "ω (Hz)"=668.1449136803938, "Γ (Hz)"=0.05932303895299783, "φ (rad)"=3.5582903583995025, "Q"=11262.823440481041, "Norm  Ampl"=0.02746775262382806, "z∞ (V)"=0.22340407289738895-0.41939959877932326i, "4corners"={"z (-pi/2)"=-0.38739959877932323-0.18340407289738891i, "z(inf)"=0.22340407289738895-0.41939959877932326i, "z (pi/2)"=0.4593995987793233+0.19140407289738892i, "z center"=0.03600000000000003+0.0040000000000000036i, "z(0)"=-0.15140407289738889+0.42739959877932326i, "radius"=0.46301998529763466}}, "timestamp(min)"=386.1499999985099, "timestamp"=timestamp(3493750990 s since 1904-01-01), "Magn Field(T)"=0.0}, {"temperature"=139.474, "lorentzian"={"A (VHz)"=0.0002528362178070129, "ω (Hz)"=668.1500479338042, "Γ (Hz)"=0.0539710421858305, "φ (rad)"=3.5123708464905583, "Q"=12379.787769027362, "Norm  Ampl"=0.0253717508779243, "z∞ (V)"=0.2063361929069562-0.43415404062471646i, "4corners"={"z (-pi/2)"=-0.40215404062471644-0.16633619290695617i, "z(inf)"=0.2063361929069562-0.43415404062471646i, "z (pi/2)"=0.4741540406247165+0.17433619290695618i, "z center"=0.03600000000000003+0.0040000000000000036i, "z(0)"=-0.13433619290695614+0.44215404062471647i, "radius"=0.4700993319818711}}, "timestamp(min)"=387.48333333432674, "timestamp"=timestamp(3493751070 s since 1904-01-01), "Magn Field(T)"=0.0}, {"temperature"=139.164, "lorentzian"={"A (VHz)"=0.0002667211730037691, "ω (Hz)"=668.1552952835116, "Γ (Hz)"=0.05603323394019338, "φ (rad)"=3.535176581973426, "Q"=11924.267944210782, "Norm  Ampl"=0.02631930849793996, "z∞ (V)"=0.21613372556427-0.4297952150996005i, "4corners"={"z (-pi/2)"=-0.3977952150996005-0.17613372556426996i, "z(inf)"=0.21613372556427-0.4297952150996005i, "z (pi/2)"=0.46979521509960054+0.18413372556426996i, "z center"=0.03600000000000003+0.0040000000000000036i, "z(0)"=-0.14413372556426993+0.4377952150996005i, "radius"=0.46970889679563493}}, "timestamp(min)"=388.80000000447035, "timestamp"=timestamp(3493751149 s since 1904-01-01), "Magn Field(T)"=0.0}, {"temperature"=138.863, "lorentzian"={"A (VHz)"=0.0002632782473768322, "ω (Hz)"=668.1649667431813, "Γ (Hz)"=0.055518318155612194, "φ (rad)"=3.5401423915730392, "Q"=12035.036163566463, "Norm  Ampl"=0.026254462824322016, "z∞ (V)"=0.21152300303333-0.43183387301036114i, "4corners"={"z (-pi/2)"=-0.4078338730103611-0.17952300303332996i, "z(inf)"=0.21152300303333-0.43183387301036114i, "z (pi/2)"=0.46383387301036116+0.18752300303332997i, "z center"=0.028000000000000025+0.0040000000000000036i, "z(0)"=-0.15552300303332994+0.43983387301036114i, "radius"=0.4728973012246774}}, "timestamp(min)"=390.1333333328366, "timestamp"=timestamp(3493751229 s since 1904-01-01), "Magn Field(T)"=0.0}, {"temperature"=138.548, "lorentzian"={"A (VHz)"=0.0002686138783751891, "ω (Hz)"=668.1727890439503, "Γ (Hz)"=0.05704297382890132, "φ (rad)"=3.58611827755777, "Q"=11713.498511632904, "Norm  Ampl"=0.027094677522831623, "z∞ (V)"=0.232258544845553-0.4248253787824388i, "4corners"={"z (-pi/2)"=-0.4008253787824388-0.20025854484555297i, "z(inf)"=0.232258544845553-0.4248253787824388i, "z (pi/2)"=0.45682537878243884+0.20825854484555298i, "z center"=0.028000000000000025+0.0040000000000000036i, "z(0)"=-0.17625854484555295+0.4328253787824388i, "radius"=0.47498711417292677}}, "timestamp(min)"=391.45000000298023, "timestamp"=timestamp(3493751308 s since 1904-01-01), "Magn Field(T)"=0.0}, {"temperature"=138.231, "lorentzian"={"A (VHz)"=0.0002580231592322443, "ω (Hz)"=668.1779102230967, "Γ (Hz)"=0.0544060199514286, "φ (rad)"=3.5599823125905723, "Q"=12281.32311129573, "Norm  Ampl"=0.02577356052556405, "z∞ (V)"=0.2204700257563606-0.4288647151278667i, "4corners"={"z (-pi/2)"=-0.4048647151278667-0.18847002575636057i, "z(inf)"=0.2204700257563606-0.4288647151278667i, "z (pi/2)"=0.46086471512786675+0.19647002575636058i, "z center"=0.028000000000000025+0.0040000000000000036i, "z(0)"=-0.16447002575636055+0.43686471512786673i, "radius"=0.4737262631703918}}, "timestamp(min)"=392.76666666567326, "timestamp"=timestamp(3493751387 s since 1904-01-01), "Magn Field(T)"=0.0}, {"temperature"=137.923, "lorentzian"={"A (VHz)"=0.00028637382702514707, "ω (Hz)"=668.1880252548099, "Γ (Hz)"=0.06079388308886444, "φ (rad)"=3.626888775238691, "Q"=10991.040402503937, "Norm  Ampl"=0.028563260628747845, "z∞ (V)"=0.24716535636177525-0.41158879722924363i, "4corners"={"z (-pi/2)"=-0.3875887972292436-0.21516535636177522i, "z(inf)"=0.24716535636177525-0.41158879722924363i, "z (pi/2)"=0.44358879722924366+0.22316535636177523i, "z center"=0.028000000000000025+0.0040000000000000036i, "z(0)"=-0.1911653563617752+0.41958879722924364i, "radius"=0.46983773987583555}}, "timestamp(min)"=394.1000000014901, "timestamp"=timestamp(3493751467 s since 1904-01-01), "Magn Field(T)"=0.0}, {"temperature"=137.615, "lorentzian"={"A (VHz)"=0.00026272492904636, "ω (Hz)"=668.192804963829, "Γ (Hz)"=0.05527490156044245, "φ (rad)"=3.5880728047733292, "Q"=12088.539031284716, "Norm  Ampl"=0.026083000913466835, "z∞ (V)"=0.2317537390572456-0.421620847218468i, "4corners"={"z (-pi/2)"=-0.39762084721846797-0.19975373905724558i, "z(inf)"=0.2317537390572456-0.421620847218468i, "z (pi/2)"=0.453620847218468+0.2077537390572456i, "z center"=0.028000000000000025+0.0040000000000000036i, "z(0)"=-0.17575373905724556+0.429620847218468i, "radius"=0.47187783563839336}}, "timestamp(min)"=395.41666666418314, "timestamp"=timestamp(3493751546 s since 1904-01-01), "Magn Field(T)"=0.0}, {"temperature"=137.3, "lorentzian"={"A (VHz)"=0.00026008216018285935, "ω (Hz)"=668.2024272814265, "Γ (Hz)"=0.0553960533268648, "φ (rad)"=3.617214392885987, "Q"=12062.274966389634, "Norm  Ampl"=0.025892490308144247, "z∞ (V)"=0.2420214777125745-0.41152845258494763i, "4corners"={"z (-pi/2)"=-0.3875284525849476-0.21002147771257448i, "z(inf)"=0.2420214777125745-0.41152845258494763i, "z (pi/2)"=0.44352845258494766+0.2180214777125745i, "z center"=0.028000000000000025+0.0040000000000000036i, "z(0)"=-0.18602147771257446+0.41952845258494764i, "radius"=0.4674067691314655}}, "timestamp(min)"=396.73333333432674, "timestamp"=timestamp(3493751625 s since 1904-01-01), "Magn Field(T)"=0.0}, {"temperature"=137.004, "lorentzian"={"A (VHz)"=0.00024818777938784227, "ω (Hz)"=668.2077960895239, "Γ (Hz)"=0.053536500417424936, "φ (rad)"=3.575640217162926, "Q"=12481.349936575929, "Norm  Ampl"=0.024927732275848467, "z∞ (V)"=0.22381537528742693-0.41844465648109325i, 
